vi "Run.vi"(8 "error in (no error)":errorcluster, 11 "DAQmx in":refnum<class "DAQmx.lvclass">) -> (0 "error out":errorcluster, 3 "DAQmx out":refnum<class "DAQmx.lvclass">)   [LabVIEW 2019, in "DAQmx.lvlib" / "DAQmx.lvclass"]
doc: "<b>Execution System:</b> Data Acquisition"
uses:
  DAQmx.lvclass
  <vilib>/DAQmx/read.llb/DAQmx Read (Analog 2D DBL NChan NSamp).vi
  <vilib>/Analysis/baseanly.llb/Mean (DBL).vi
  <vilib>/DAQmx/read.llb/DAQmx Read (Digital 1D Bool NChan 1Samp 1Line).vi
  <vilib>/DAQmx/miscellaneous.llb/DAQmx Fill In Error Info.vi
  <vilib>/Analysis/NI_AALBase.lvlib
  Plugin Interfaces/Controller Interface/Controller Interface.lvlibp/Controller Interface Class/Controller Interface.lvclass
  C:/github/dataflowg/dataflow-dj/src/Plugin Interfaces/Controller Interface/Controller Interface.lvlibp/Controller Interface Class/Controller Interface.lvclass
panel:
  out "DI Error":errorcluster
  out "AI Error":errorcluster
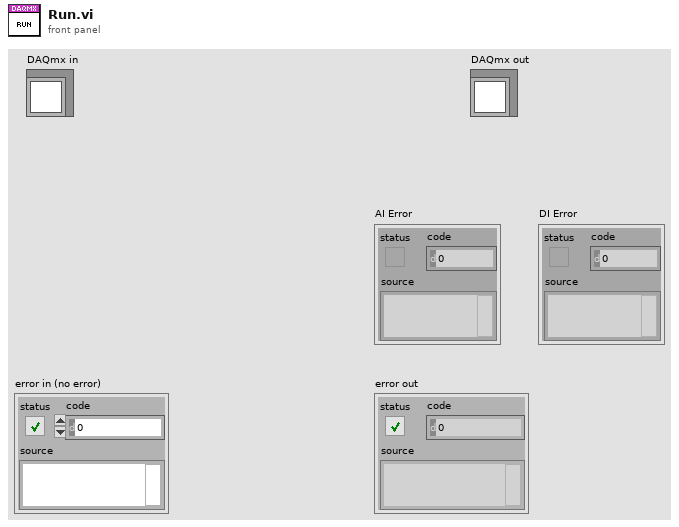
[diagram p1: front panel]
types:
  T1 = typedef "DAQmx.lvlib/DAQmx.lvclass/DAQmx Shortcut.ctl" = cluster{"DAQmx Global Channel":refnum<k21>, "Message Queue":string, "Event":string, "Target":string, "Momentary":bool, "Data":variant}
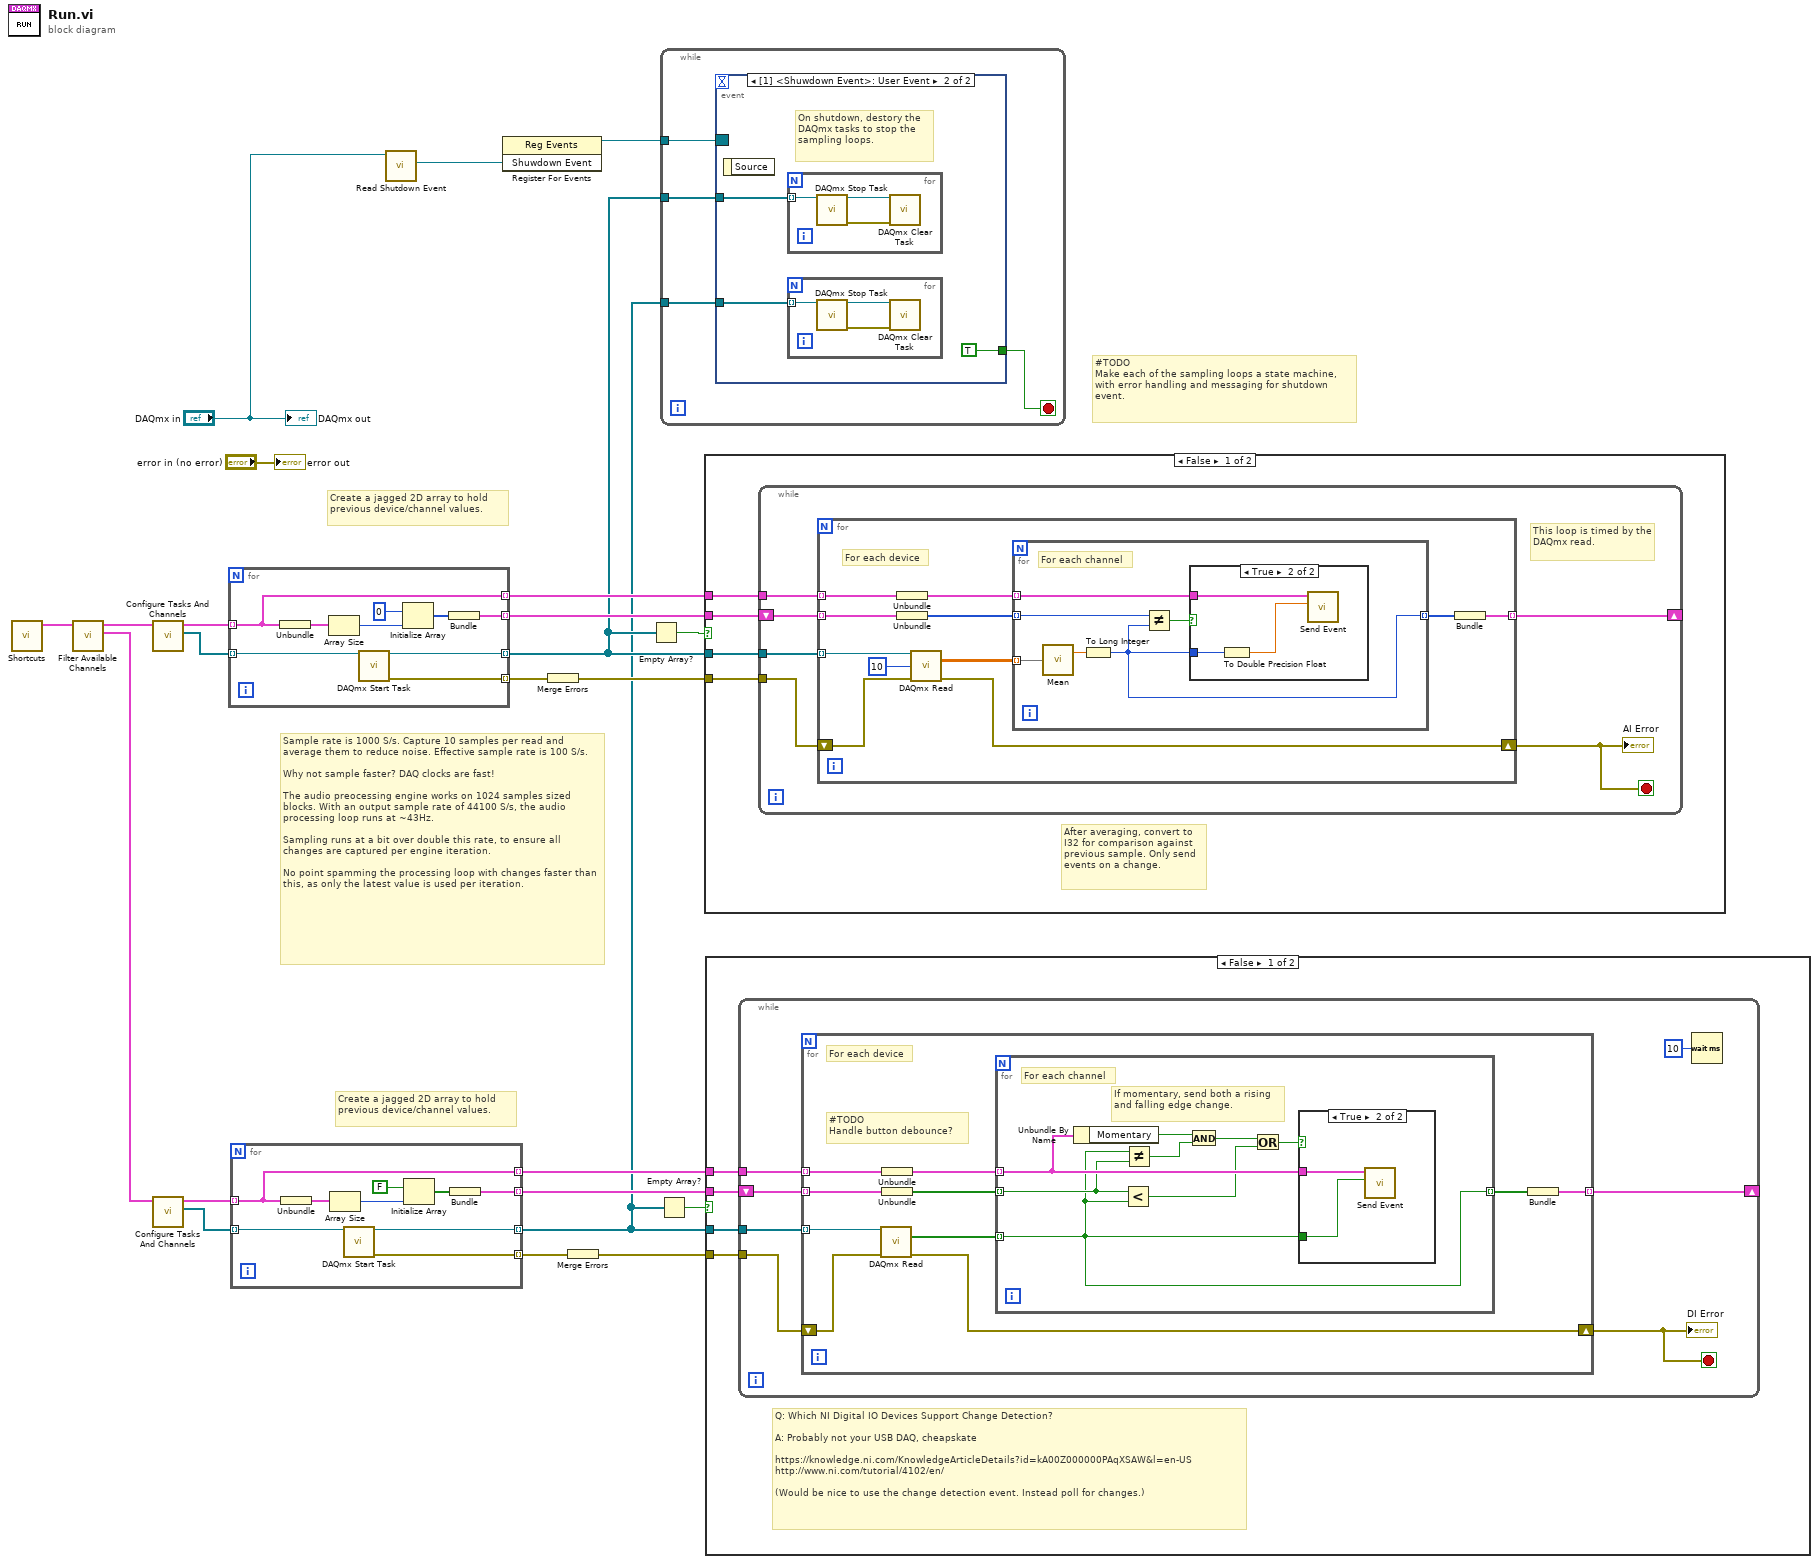
[diagram p0: block diagram]
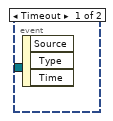
[diagram p6: hidden frame]
diagram:
  # "#TODO\nMake each of the sampling loops a state machine, with error handling and messaging for shutdown event."
  # "Create a jagged 2D array to hold previous device/channel values."
  # "Create a jagged 2D array to hold previous device/channel values."
  # "Sample rate is 1000 S/s. Capture 10 samples per read and average them to reduce noise. Effective sample rate is 100 S/s.\n\nWhy not sample faster? DAQ clocks are fast!\n\nThe audio preocessing engine works on 1024 samples sized blocks. With an output sample rate of 44100 S/s, the audio processing loop runs at ~43Hz.\n\nSampling runs at a bit over double this rate, to ensure all changes are captured per engine iteration.\n\nNo point spamming the processing loop with changes faster than this, as only the latest value is used per iteration."
  n1 = call "Shortcuts.vi"() -> ("DAQmx Shortcuts"=w3:T1[])  [unwired: 11 in]
  n2 = call "Filter Available Channels.vi"("DAQmx Shortcuts"=w3) -> ("DAQmx DI Shortcuts"=w18:T1[], "DAQmx AI Shortcuts"=w19:T1[])  [unwired: 9 in]
  n3 = call "Configure Tasks And Channels.vi"("DAQmx Shortcuts"=w19) -> ("Task Per Device"=w16:refnum<k21>[], "DAQmx Shortcuts Per Device"=w17:cluster{T1[]}[])  [unwired: 9 in]
  n4 = call "Configure Tasks And Channels.vi"("DAQmx Shortcuts"=w18) -> ("Task Per Device"=w14:refnum<k21>[], "DAQmx Shortcuts Per Device"=w15:cluster{T1[]}[])  [unwired: 9 in]
  n5 = for {
    tunnel: [w32] -> w23 mode=indexing
    tunnel: [w31] -> w22 mode=indexing
    tunnel: [w30] -> w8 mode=indexing
    tunnel: w16 -> [w29] mode=indexing
    tunnel: w17 -> [w24] mode=indexing
    tunnel: [w24] -> w20 mode=indexing
    n6 = Unbundle(w24) -> (w25:T1[])
    n7 = Array Size(array=w25) -> (size(s)=w27:i32)
    n8 = call <vilib>:"DAQmx Start Task.vi"("task/channels in"=w29) -> ("task out"=w30:refnum<k21>, "error out"=w32:errorcluster)  [unwired: 13 in]
    n9 = Initialize Array(0 ("element"), w27) -> (w26:i32[])
    n10 = Bundle(w26) -> (w31:cluster{i32[]})  [unwired: 1 in]
  }
  n11 = for {
    tunnel: [w41] -> w13 mode=indexing
    tunnel: [w40] -> w11 mode=indexing
    tunnel: [w39] -> w6 mode=indexing
    tunnel: w14 -> [w38] mode=indexing
    tunnel: w15 -> [w33] mode=indexing
    tunnel: [w33] -> w10 mode=indexing
    n12 = Unbundle(w33) -> (w34:T1[])
    n13 = Array Size(array=w34) -> (size(s)=w36:i32)
    n14 = call <vilib>:"DAQmx Start Task.vi"("task/channels in"=w38) -> ("task out"=w39:refnum<k21>, "error out"=w41:errorcluster)  [unwired: 13 in]
    n15 = Initialize Array(FALSE, w36) -> (w35:bool[])
    n16 = Bundle(w35) -> (w40:cluster{bool[]})  [unwired: 1 in]
  }
  n17 = call "Read Shutdown Event.vi"("Controller Interface in"="DAQmx in") -> ("Shuwdown Event"=w1:refnum<user-event>)  [unwired: 9 in, 1 out]
  n18 = register-events(w1) -> (reference out=w21:refnum<event-registration>)  [unwired: 2 in, 1 out]
  n19 = Merge Errors(w23) -> (w9:errorcluster)
  n20 = Merge Errors(w13) -> (w12:errorcluster)
  n21 = Empty Array?(array=w8) -> (empty?=w7:bool)
  n22 = Empty Array?(array=w6) -> (empty?=w5:bool)
  n23 = while {
    tunnel: w21 -> [w45]
    tunnel: w8 -> [w43]
    tunnel: w6 -> [w42]
    stop <- w44 stop-if-true
    n24 = event shown="[1] <Shuwdown Event>: User Event" {
      selector: w45 -> [_ _]
      dyn-events: _ -> [_ _]
      timeout: _ -> [_ _]
      tunnel: [_ TRUE] -> w44
      tunnel: w43 -> [_ w47]
      tunnel: w42 -> [_ w46]
      event Timeout {
        n25 = event-data() -> ()  [unwired: 1 in, 3 out]
      }
      event User Event {
        # "On shutdown, destory the DAQmx tasks to stop the sampling loops."
        n26 = event-data() -> ()  [unwired: 1 in, 1 out]
        n27 = for {
          tunnel: w47 -> [w52] mode=indexing
          n28 = call <vilib>:"DAQmx Stop Task.vi"("task/channels in"=w52) -> ("task out"=w53:refnum<k21>, "error out"=w54:errorcluster)  [unwired: 13 in]
          n29 = call <vilib>:"DAQmx Clear Task.vi"("task in"=w53, "error in"=w54) -> ()  [unwired: 13 in, 1 out]
        }
        n30 = for {
          tunnel: w46 -> [w49] mode=indexing
          n31 = call <vilib>:"DAQmx Stop Task.vi"("task/channels in"=w49) -> ("task out"=w50:refnum<k21>, "error out"=w51:errorcluster)  [unwired: 13 in]
          n32 = call <vilib>:"DAQmx Clear Task.vi"("task in"=w50, "error in"=w51) -> ()  [unwired: 13 in, 1 out]
        }
      }
    }
  }
  n33 = case shown="False" w7 {
    tunnel: w22 -> [w58 _]
    tunnel: w20 -> [w57 _]
    tunnel: w9 -> [w56 _]
    tunnel: w8 -> [w55 _]
    frame False {
      # "After averaging, convert to I32 for comparison against previous sample. Only send events on a change."
      n34 = while {
        tunnel: w55 -> [w64]
        tunnel: w56 -> [w63]
        tunnel: w57 -> [w61]
        shift-right: [w60] -> _
        shift-left: w58 -> [w62]
        stop <- w59 stop-if-true
        # "This loop is timed by the DAQmx read."
        n35 = for {
          tunnel: w64 -> [w75] mode=indexing
          tunnel: w62 -> [w67] mode=indexing
          tunnel: w61 -> [w71] mode=indexing
          tunnel: [w65] -> w60 mode=indexing
          shift-right: [w69] -> w59
          shift-left: w63 -> [w74]
          # "For each device"
          n36 = Unbundle(w71) -> (w66:T1[])
          n37 = Unbundle(w67) -> (w68:i32[])
          n38 = call-poly <vilib>:"DAQmx Read.vi"("task/channels in"=w75, "number of samples per channel"=10, "error in"=w74) -> ("data"=w72:dbl[][], "error out"=w69:errorcluster)  [unwired: 10 in, 1 out]
          n39 = for {
            tunnel: w72 -> [w81] mode=indexing
            tunnel: w68 -> [w80] mode=indexing
            tunnel: w66 -> [w79] mode=indexing
            tunnel: [w76] -> w70 mode=indexing
            # "For each channel"
            n40 = call-poly <vilib>:"Mean.vi"("X"=w81) -> ("mean"=w77:dbl)  [unwired: 1 out]
            n41 = To Long Integer(number=w77) -> (32bit integer=w76:i32)
            n42 = Not Equal?(x=w80, y=w76) -> (x != y?=w78:bool)
            n43 = case shown="True" w78 {
              tunnel: w79 -> [_ w83]
              tunnel: w76 -> [_ w84]
              frame False {
              }
              frame True {
                n44 = To Double Precision Float(number=w84) -> (double precision float=w82:dbl)
                n45 = call "Send Event.vi"("Data"=w82, "DAQmx Shortcut"=w83) -> ()  [unwired: 10 in]
              }
            }
          }
          n46 = Bundle(w70) -> (w65:cluster{i32[]})  [unwired: 1 in]
        }
        "AI Error" <- w59
      }
    }
    frame True {
    }
  }
  n47 = case shown="False" w5 {
    tunnel: w12 -> [w88 _]
    tunnel: w6 -> [w87 _]
    tunnel: w11 -> [w86 _]
    tunnel: w10 -> [w85 _]
    frame False {
      # "Q: Which NI Digital IO Devices Support Change Detection?\n\nA: Probably not your USB DAQ, cheapskate\n\nhttps://knowledge.ni.com/KnowledgeArticleDetails?id=kA00Z000000PAqXSAW&l=en-US\nhttp://www.ni.com/tutorial/4102/en/\n\n(Would be nice to use the change detection event. Instead poll for changes.)"
      n48 = while {
        tunnel: w88 -> [w93]
        tunnel: w87 -> [w94]
        tunnel: w85 -> [w91]
        shift-right: [w90] -> _
        shift-left: w86 -> [w92]
        stop <- w89 stop-if-true
        n49 = for {
          tunnel: w94 -> [w105] mode=indexing
          tunnel: w92 -> [w101] mode=indexing
          tunnel: w91 -> [w102] mode=indexing
          tunnel: [w96] -> w90 mode=indexing
          shift-right: [w98] -> w89
          shift-left: w93 -> [w104]
          # "#TODO\nHandle button debounce?"
          # "For each device"
          n50 = call-poly <vilib>:"DAQmx Read.vi"("task/channels in"=w105, "error in"=w104) -> ("data"=w103:bool[], "error out"=w98:errorcluster)  [unwired: 11 in, 1 out]
          n51 = Unbundle(w102) -> (w100:T1[])
          n52 = Unbundle(w101) -> (w99:bool[])
          n53 = for {
            tunnel: w103 -> [w108] mode=indexing
            tunnel: w100 -> [w112] mode=indexing
            tunnel: w99 -> [w109] mode=indexing
            tunnel: [w108] -> w97 mode=indexing
            # "If momentary, send both a rising and falling edge change."
            # "For each channel"
            n54 = Unbundle By Name(w112) -> ("Momentary"=w111:bool)
            n55 = Less?(x=w109, y=w108) -> (x < y?=w107:bool)
            n56 = Not Equal?(x=w108, y=w109) -> (x != y?=w113:bool)
            n57 = And(x=w111, y=w113) -> (x .and. y?=w110:bool)
            n58 = Or(x=w110, y=w107) -> (x .or. y?=w106:bool)
            n59 = case shown="True" w106 {
              tunnel: w112 -> [_ w115]
              tunnel: w108 -> [_ w114]
              frame False {
              }
              frame True {
                n60 = call "Send Event.vi"("Data"=w114, "DAQmx Shortcut"=w115) -> ()  [unwired: 10 in]
              }
            }
          }
          n61 = Bundle(w97) -> (w96:cluster{bool[]})  [unwired: 1 in]
        }
        "DI Error" <- w89
        n62 = Wait (ms)(milliseconds to wait=u32 10) -> ()  [unwired: 1 out]
      }
    }
    frame True {
    }
  }
  "error out" <- "error in (no error)"
  "DAQmx out" <- "DAQmx in"
